vi "Disabled - Read File into 1D Array (SubVI).vi"(4 "Reload":bool, 5 "Path":string="/c/tmp/auton/", 6 "error in":errorcluster, 7 "File Name":string="test.pi") -> (0 "all rows":dbl[][](array[numeric]), 1 "error out":errorcluster, 3 "File Name":string="test.pi")   [LabVIEW 2020]
uses:
  <vilib>/Utility/file.llb/Read Delimited Spreadsheet (DBL).vi
panel:
  # "Load Auton File Into Array"
  # "Inputs"
  # "Outputs"
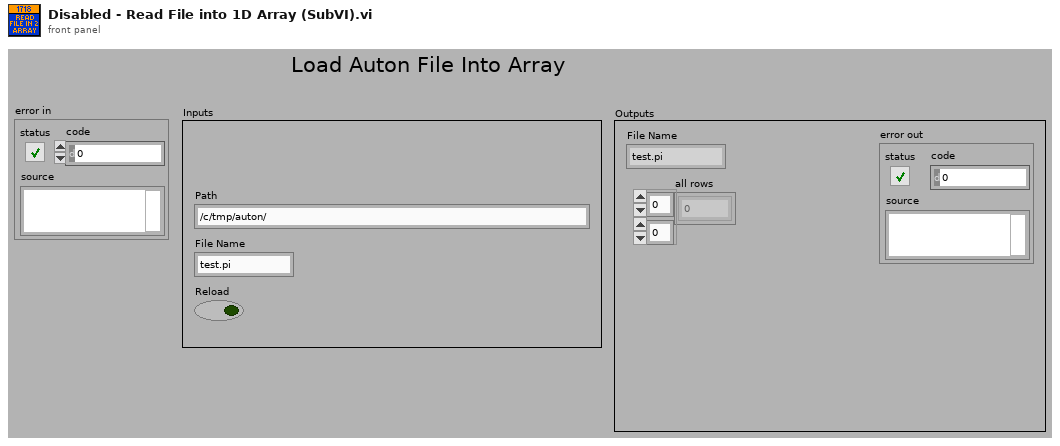
[diagram p1: front panel]
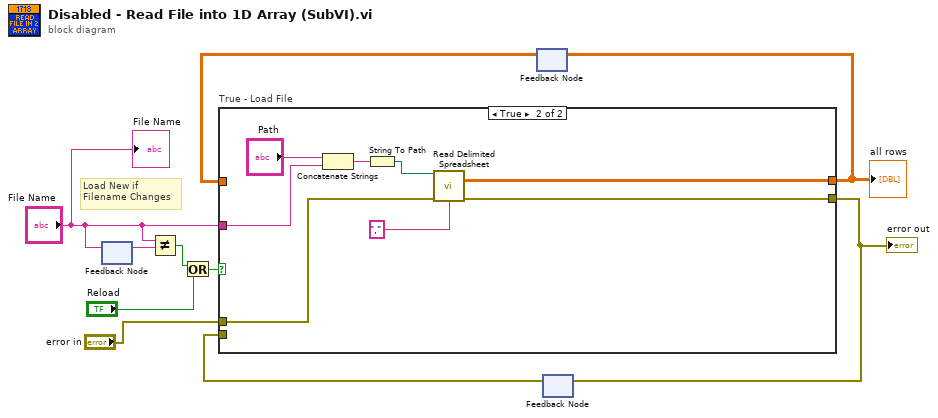
[diagram p0: block diagram]
diagram:
  # "Load New if\nFilename Changes"
  n1 = feedback-in #1("File Name") -> ()
  n2 = feedback #1() -> (w8:string)  [unwired: 1 in]
  n3 = Not Equal?(x="File Name", y=w8) -> (x != y?=w6:bool)
  n4 = Or(x=w6, y="Reload") -> (x .or. y?=w7:bool)
  n5 = feedback #2() -> (w10:dbl[][])  [unwired: 1 out]
  n6 = feedback #3() -> (w2:errorcluster)  [unwired: 1 out]
  n7 = case "True - Load File" shown="True" w7 {
    tunnel: [w12 w15] -> w4
    tunnel: w10 -> [w12 _]
    tunnel: "File Name" -> [_ w18]
    tunnel: [w11 w14] -> w3
    tunnel: w2 -> [w11 _]
    tunnel: "error in" -> [_ w13]
    frame False {
    }
    frame True {
      n8 = Concatenate Strings "Concatenate Strings"("Path", w18) -> (w20:string)
      n9 = String To Path(string=w20) -> (path=w16:path)
      n10 = call-poly <vilib>:"Read Delimited Spreadsheet.vi"("file path (dialog if empty)"=w16, "error in (no error)"=w13, "delimiter (\\t)"="," ("delimiter (\\t)")) -> ("all rows"=w15:dbl[][], "error out"=w14:errorcluster)  [unwired: 7 in, 4 out]
    }
  }
  "all rows" <- w4
  "error out" <- w3
  n11 = feedback-in #2(w4) -> ()
  n12 = feedback-in #3(w3) -> ()
  "File Name" <- "File Name"
